vi "test Thermal Chamber Response Simulator_Init-Error Before Init.vi"(8 "error in (no error)":errorcluster, 11 "TestCase in":refnum<class "Thermal Chamber Response Simulator_Init.lvclass">) -> (0 "error out":errorcluster, 3 "TestCase out":refnum<class "Thermal Chamber Response Simulator_Init.lvclass">)   [LabVIEW 2018, in "Thermal Chamber Response Simulator_Init.lvclass"]
uses:
  Thermal Chamber Response Simulator_Init.lvclass
  Libraries/Thermal Chamber Response Simulator/Thermal Chamber Response Simulator.lvlib
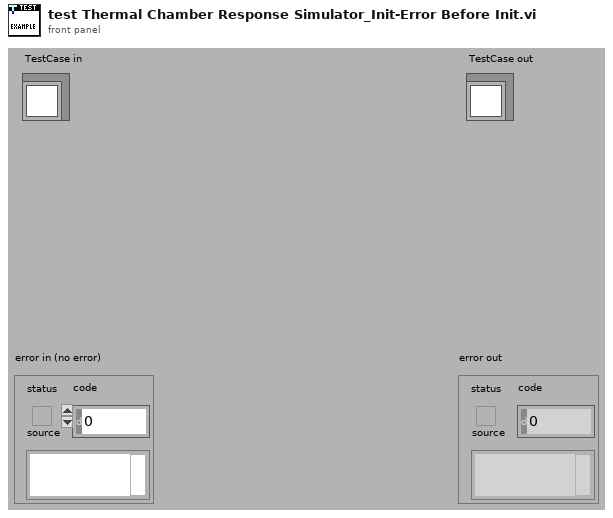
[diagram p1: front panel]
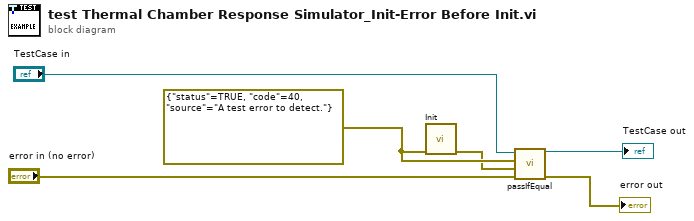
[diagram p0: block diagram]
diagram:
  w6 = errorcluster {"status"=TRUE, "code"=40, "source"="A test error to detect."} ("error out")
  n1 = call "Init.vi"("error in (no error)"=w6) -> ("error out"=w5:errorcluster)  [unwired: 10 in]
  n2 = call-dynamic "passIfEqual.vi"("error in (no error)"="error in (no error)", "y"=w5, "x"=w6, "TestCase in"="TestCase in") -> ("error out"=→"error out":errorcluster, "TestCase out"=→"TestCase out":refnum<class "Thermal Chamber Response Simulator_Init.lvclass">)  [unwired: 6 in]
